vi "CatchError.vi"(8 "error in (no error)":errorcluster, 11 "Logger in":refnum<class "Logger.lvclass">) -> (0 "error out":errorcluster, 3 "Logger out":refnum<class "Logger.lvclass">)   [LabVIEW 2026, in "Lumberjack.lvlib" / "Logger.lvclass"]
doc: "Catches an incoming error, logs it at ERROR, and optionally surfaces it to the operator.\nIf error in carries an error, builds an ERROR-level Statement from it and enqueues it through the resolved logger, then clears the error so the caller continues; whether the General Error Handler dialog is shown is gated by the process CatchError verbosity (GetVerbosity + ShouldDisplay). No-op passthrough on no error or if no logger resolves.\nLumberjack.lvlib, Logger.lvclass, public."
uses:
  Logger.lvclass
  TypeDefs/Severity.ctl
  Lumberjack.lvlib
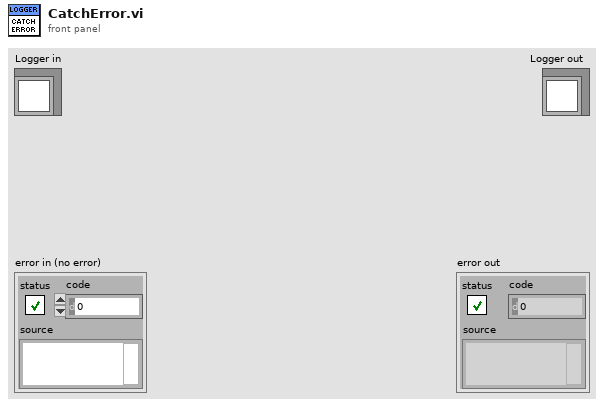
[diagram p1: front panel]
types:
  T1 = typedef "Lumberjack.lvlib/Severity.ctl" = enum16{"OFF", "FATAL", "ERROR", "WARN", "INFO", "DEBUG", "TRACE", "ALL"}
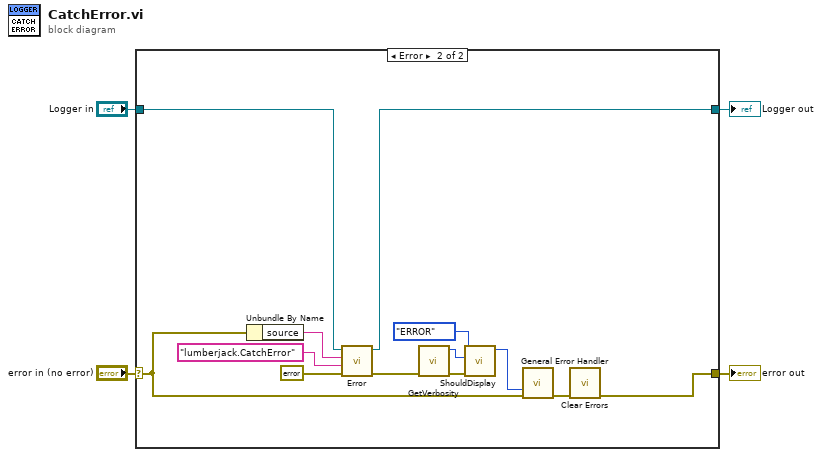
[diagram p0: block diagram]
diagram:
  n1 = case shown="Error" "error in (no error)" {
    selector: "error in (no error)" -> [w5 w9]
    tunnel: [w5 w7] -> w3
    tunnel: [w6 w15] -> w1
    tunnel: "Logger in" -> [w6 w19]
    frame No Error {
      # "Wire the error cluster across even in the \"No Error\"\ncase so that warnings get propagated."
    }
    frame Error {
      n2 = Unbundle By Name(w9) -> ("source"=w18:string)
      n3 = call "Error.vi"("error in (no error)"=errorcluster {"status"=FALSE, "code"=0, "source"=""} ("error out"), "sourceTag"="lumberjack.CatchError", "message"=w18, "Logger in"=w19) -> ("error out"=w16:errorcluster, "Logger out"=w15:refnum<class "Logger.lvclass">)  [unwired: 6 in]
      n4 = call "GetVerbosity.vi"("error in (no error)"=w16) -> ("error out"=w12:errorcluster, "Verbosity"=w13:T1)  [unwired: 8 in, 1 out]
      n5 = call "ShouldDisplay.vi"("error in (no error)"=w12, "verbosity"=w13, "errorSeverity"=Severity."ERROR" ("Level")) -> ("dialogType"=w10:i32)  [unwired: 7 in, 1 out]
      n6 = call <vilib>:"General Error Handler.vi"("type of dialog (OK msg:1)"=w10, "error in (no error)"=w9) -> ("error out"=w8:errorcluster)  [unwired: 9 in, 4 out]
      n7 = call <vilib>:"Clear Errors.vi"("error in (no error)"=w8) -> ("error out"=w7:errorcluster)  [unwired: 5 in, 1 out]
    }
  }
  "error out" <- w3
  "Logger out" <- w1
